vi "Pre-Init.vi"(8 "error in (no error)":errorcluster, 11 "Pulse Driver in":refnum<class "Pulse Driver.lvclass">) -> (0 "error out":errorcluster, 3 "Pulse Driver out":refnum<class "Pulse Driver.lvclass">)   [LabVIEW 2021, in "Pulse Driver.lvclass"]
uses:
  Pulse Driver.lvclass
  C:/GitHub/NHMFL_Core/Libraries/Instruments/Instrument Driver/Instrument Driver.lvclass
  Instrument Driver/Instrument Driver.lvclass/Instrument Driver.ctl
  Pulse Driver.lvclass/Pulse Driver.ctl
  177aa3ad-ceef-4f55-896b-3dd49bc0a2ae.vi
  Instrument Driver/Read Recorder name.vi
  Write Samples per channel.vi
  Write Pretrigger samples.vi
  Instrument Driver/Write Channel names.vi
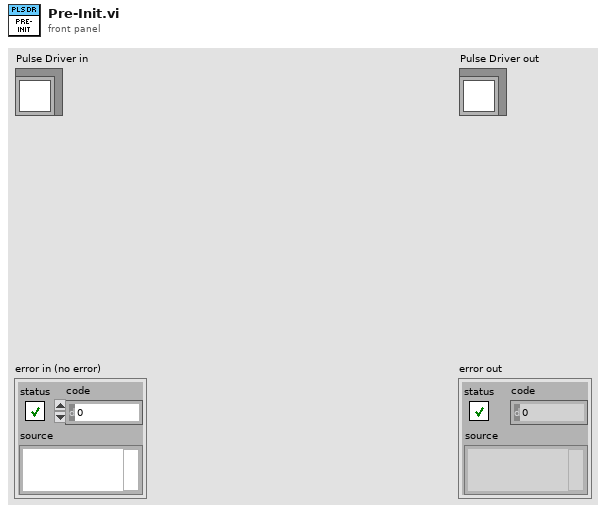
[diagram p1: front panel]
types:
  T1 = typedef "Pusle Driver Configuration.ctl" = cluster{"Post-trigger delay":dbl, "Post-trigger duration":dbl, "Rate":dbl, "Ranges":dbl[], "Re-name channels":string[], "Active channels":string, "External clock":bool}
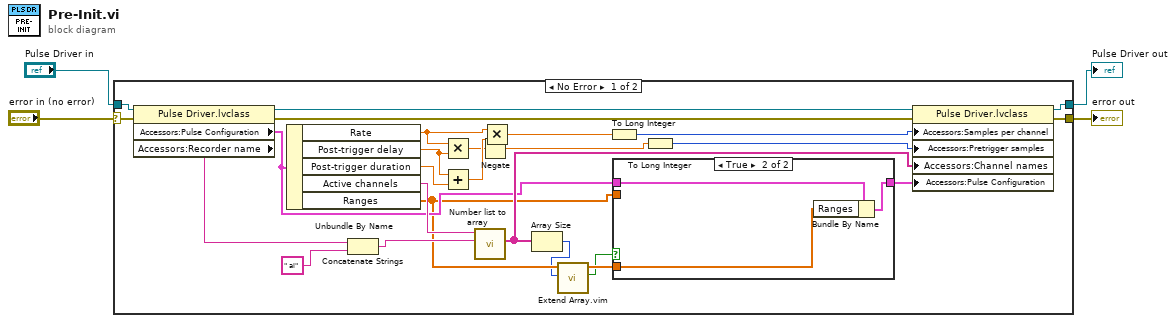
[diagram p0: block diagram]
diagram:
  n1 = case shown="No Error" "error in (no error)" {
    selector: "error in (no error)" -> [w18 w36]
    tunnel: [w17 w36] -> w3
    tunnel: [w27 w35] -> w1
    tunnel: "Pulse Driver in" -> [w30 w35]
    frame No Error {
      n2 = property class="Pulse Driver.lvclass"(reference=w30, error in=w18) -> (reference out=w29:refnum<class "Pulse Driver.lvclass">, error out=w19:errorcluster, "Accessors:Pulse Configuration"=w14:T1, "Accessors:Recorder name"=w12:string)
      n3 = Unbundle By Name(w14) -> ("Rate"=w20:dbl, "Post-trigger delay"=w23:dbl, "Post-trigger duration"=w28:dbl, "Active channels"=w16:string, "Ranges"=w9:dbl[])
      n4 = Concatenate Strings(w12, " ai" ("Full names prefix")) -> (w10:string)
      n5 = Multiply(x=w20, y=w23) -> (x*y=w22:dbl)
      n6 = Add(x=w23, y=w28) -> (x+y=w25:dbl)
      n7 = call "Number list to array.vi"("Full names prefix"=w10, "Number list"=w16) -> ("Full names"=w15:string[])  [unwired: 8 in, 1 out]
      n8 = Negate(x=w22) -> (-x=w5:dbl)
      n9 = Multiply(x=w20, y=w25) -> (x*y=w24:dbl)
      n10 = Array Size(array=w15) -> (size(s)=w8:i32)
      n11 = call "Extend Array.vim"("Extend to size"=w8, "Array in"=w9) -> ("Extended"=w6:bool, "Array out"=w7:dbl[])  [unwired: 8 in]
      n12 = To Long Integer(number=w24) -> (32bit integer=w26:i32)
      n13 = case shown="True" w6 {
        tunnel: w9 -> [_ _]
        tunnel: w14 -> [w31 w34]
        tunnel: [w31 w33] -> w13
        tunnel: w7 -> [_ w32]
        frame False {
        }
        frame True {
          n14 = Bundle By Name(cluster=w34, "Ranges"=w32) -> (w33:T1)
        }
      }
      n15 = To Long Integer(number=w5) -> (32bit integer=w21:i32)
      n16 = property class="Pulse Driver.lvclass"(reference=w29, error in=w19, "Accessors:Samples per channel"=w26, "Accessors:Pretrigger samples"=w21, "Accessors:Channel names"=w15, "Accessors:Pulse Configuration"=w13) -> (reference out=w27:refnum<class "Pulse Driver.lvclass">, error out=w17:errorcluster)
    }
    frame Error {
    }
  }
  "error out" <- w3
  "Pulse Driver out" <- w1
